vi "CRC-8-CCITT.vi"(0 "CRC In":u8 format="%.0x", 5 "Reset":bool, 7 "Data":u8 format="%.0x", 11 "error in (no error)":errorcluster) -> (4 "CRC":u8 format="%.0x", 15 "error out":errorcluster)   [LabVIEW 2012]
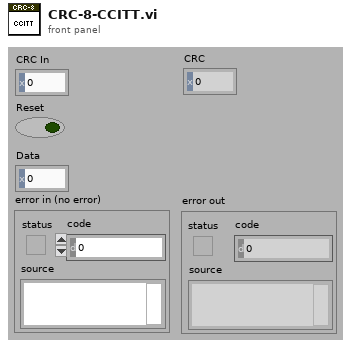
[diagram p1: front panel]
types:
  T1 = enum16{"CRC-8-CCITT", "CRC-8-Maxim 1-Wire (DOW)"}
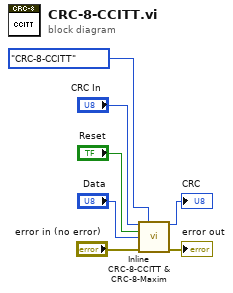
[diagram p0: block diagram]
diagram:
  n1 = call "Inline CRC-8-CCITT & CRC-8-Maxim.vi"("CRC In"="CRC In", "CRC-8 Type"=T1."CRC-8-CCITT", "Reset"="Reset", "Data"="Data", "error in (no error)"="error in (no error)") -> ("CRC"=→"CRC":u8, "error out"=→"error out":errorcluster)  [unwired: 9 in]
